vi "RSZVB Get Virtual Transform Ground Loop Circuit Model.vi"(8 "error in (no error)":errorcluster {"code" format="%.0x"}, 9 "Function Type (0)":i32(ring) items=["Deembedding", "Embedding"], 10 "Channel (1)":i32=1, 11 "VISA session":refnum<visa-resource-name>) -> (0 "error out":errorcluster {"code" format="%.0x"}, 1 "Circuit Model":i32, 3 "dup VISA session":refnum<visa-resource-name>)   [LabVIEW 2011]
doc: "This VI returns the circuit model for ground loop deembedding/embedding.\n\nRemote-control command(s):\nCALCulate<Ch>:TRANsform:VNETworks:GLOop:DEEMbedding:TNDefinition? \nCALCulate<Ch>:TRANsform:VNETworks:GLOop:EMBedding:TNDefinition?"
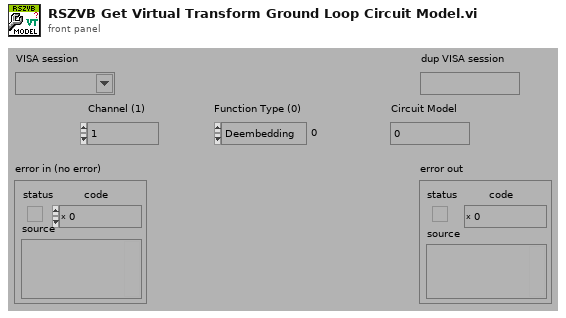
[diagram p1: front panel]
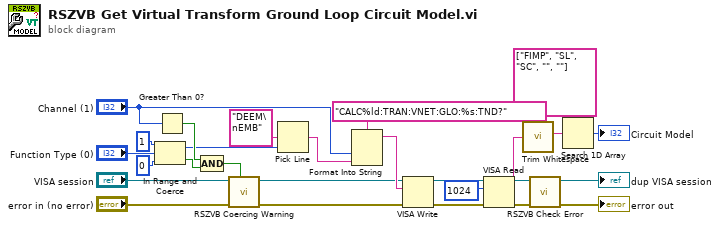
[diagram p0: block diagram]
diagram:
  n1 = In Range and Coerce(upper limit=1, x="Function Type (0)", lower limit=0) -> (coerced(x)=w13:i32, In Range?=w25:bool)
  n2 = Greater Than 0?(x="Channel (1)") -> (x > 0?=w26:bool)
  n3 = Compound Arithmetic op=AND(w26, w25) -> (w27:bool)
  n4 = call "RSZVB Coercing Warning.vi"("In Range?"=w27, "error in (no error)"="error in (no error)", "VISA session"="VISA session") -> ("error out"=w19:errorcluster, "dup VISA session"=w18:refnum<visa-resource-name>)  [unwired: 7 in]
  n5 = Pick Line(multi-line string="DEEM\nEMB", line index=w13) -> (output string=w24:string)  [unwired: 1 in]
  n6 = Format Into String(format string="CALC%ld:TRAN:VNET:GLO:%s:TND?", "Channel (1)", w24) -> (resulting string=w20:string)  [unwired: 2 in, 1 out]
  n7 = VISA Write(VISA resource name=w18, write buffer=w20, error in (no error)=w19) -> (VISA resource name out=w5:refnum<visa-resource-name>, error out=w4:errorcluster)  [unwired: 1 out]
  n8 = VISA Read(VISA resource name=w5, byte count=u32 1024 ("byte count (0)"), error in (no error)=w4) -> (VISA resource name out=w10:refnum<visa-resource-name>, read buffer=w6:string, error out=w9:errorcluster)  [unwired: 1 out]
  n9 = call <vilib>:"Trim Whitespace.vi"("string"=w6) -> ("trimmed string"=w8:string)  [unwired: 1 in]
  n10 = call "RSZVB Check Error.vi"("error in (no error)"=w9, "VISA session"=w10) -> ("error out"=→"error out":errorcluster, "dup VISA session"=→"dup VISA session":refnum<visa-resource-name>)  [unwired: 8 in]
  n11 = Search 1D Array(1D array=string[] ["FIMP", "SL", "SC", "", ""] ("array 2"), element=w8) -> (index of element=→"Circuit Model":i32)  [unwired: 1 in]
